vi "iRobot UART Close.vi"(8 "error in":errorcluster, 11 "UART port in":T1) -> (0 "error out":errorcluster)   [LabVIEW 2013]
doc: "Closes the UART port connected to iRobot. The port must be reinitialized before reuse."
uses:
  iRobot UART Port Type.ctl
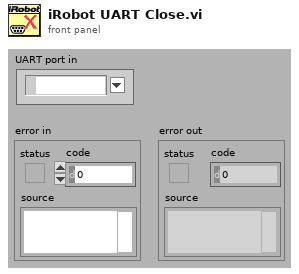
[diagram p1: front panel]
types:
  T1 = typedef "iRobot UART Port Type.ctl" = refnum<visa-resource-name>
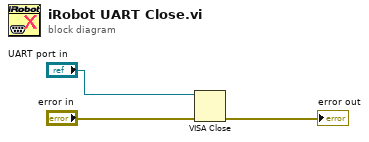
[diagram p0: block diagram]
diagram:
  n1 = VISA Close(VISA resource name="UART port in", error in (no error)="error in") -> (error out=→"error out":errorcluster)
